vi "DualMotor.vi"(10 "Speed-R":i8(knob) min=-100 max=100 step=1 scale=-100.0..100.0, 11 "Speed-L":i8(knob) min=-100 max=100 step=1 scale=-100.0..100.0) -> ()   [LabVIEW 2017]
uses:
  <vilib>/myRIO/Instrument Drivers/Onboard IO/UART/typedef/VISA Configuration.ctl
  <vilib>/Instr/_visa.llb/VISA Configure Serial Port (Instr).vi
  <vilib>/myRIO/Express VI/Onboard IO/UART/UART Express VI.xnode
  <vilib>/myRIO/Instrument Drivers/Onboard IO/UART/UART.lvlib
panel:
  out "Pololu PWM Value 2":u8
  out "Pololu PWM Value":u8
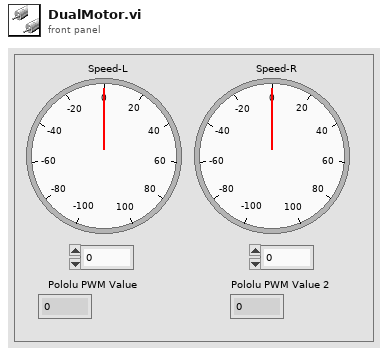
[diagram p1: front panel]
types:
  T1 = typedef "UART.lvlib/VISA Configuration.ctl" = cluster{"baud rate (9600)":u32, "data bits (8)":u16, "parity (0:none)":enum16{"None", "Odd", "Even", "Mark", "Space"}, "stop bits (10: 1 bit)":u16, "flow control (0:none)":u16, "termination char\n(0xA = '\\n' = LF) ":u8, "Enable Termination\nChar (T)":bool, "timeout (10sec)":u32}
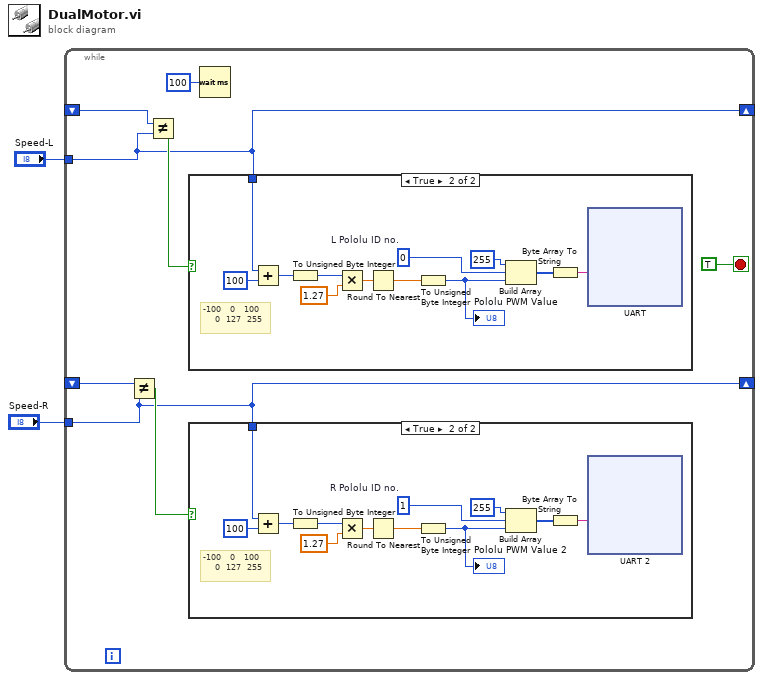
[diagram p0: block diagram]
diagram:
  n1 = while {
    shift-right: [w7] -> _
    shift-left: _ -> [w9]
    tunnel: "Speed-L" -> [w7]
    tunnel: "Speed-R" -> [w4]
    shift-right: [w4] -> _
    shift-left: _ -> [w6]
    stop <- TRUE stop-if-true
    n2 = Not Equal?(x=w6, y=w4) -> (x != y?=w5:bool)
    n3 = Not Equal?(x=w9, y=w7) -> (x != y?=w8:bool)
    n4 = case shown="True" w8 {
      tunnel: w7 -> [_ w39]
      frame False {
      }
      frame True {
        w49 = u8 0  # L Pololu ID no.
        # "-100   0   100\n    0  127  255"
        n5 = Add(x=w39, y=i8 100) -> (x+y=w41:i8)
        n6 = To Unsigned Byte Integer(number=w41) -> (unsigned 8bit integer=w40:u8)
        n7 = Multiply(x=w40, y=1.27) -> (x*y=w44:dbl)
        n8 = Round To Nearest(number=w44) -> (nearest integer value=w43:dbl)
        n9 = To Unsigned Byte Integer(number=w43) -> (unsigned 8bit integer=w45:u8)
        "Pololu PWM Value" <- w45
        n10 = Build Array(u8 255 ("element"), w49, w45) -> (w46:u8[])
        n11 = Byte Array To String(unsigned byte array=w46) -> (string=w47:string)
        n12 = xnode "UART"("Characters to Write"=w47) -> ()  [unwired: 1 in, 2 out]
      }
    }
    n13 = case shown="True" w5 {
      tunnel: w4 -> [_ w11]
      frame False {
      }
      frame True {
        w21 = u8 1  # R Pololu ID no.
        # "-100   0   100\n    0  127  255"
        n14 = Add(x=w11, y=i8 100) -> (x+y=w13:i8)
        n15 = To Unsigned Byte Integer(number=w13) -> (unsigned 8bit integer=w12:u8)
        n16 = Multiply(x=w12, y=1.27) -> (x*y=w16:dbl)
        n17 = Round To Nearest(number=w16) -> (nearest integer value=w15:dbl)
        n18 = To Unsigned Byte Integer(number=w15) -> (unsigned 8bit integer=w17:u8)
        "Pololu PWM Value 2" <- w17
        n19 = Build Array(u8 255 ("element"), w21, w17) -> (w18:u8[])
        n20 = Byte Array To String(unsigned byte array=w18) -> (string=w19:string)
        n21 = xnode "UART 2"("Characters to Write"=w19) -> ()  [unwired: 1 in, 2 out]
      }
    }
    n22 = Wait (ms)(milliseconds to wait=u32 100) -> ()  [unwired: 1 out]
  }
